vi "SPI peripheral1.vi"() -> ()   [LabVIEW 2014]
uses:
  <vilib>/Platform/TimedLoop/XDataNode/timing_clust.ctl
  <vilib>/Platform/TimedLoop/XDataNode/nitl_modes.ctl
  <vilib>/Platform/TimedLoop/XDataNode/wakeup.ctl
  <userlib>/_NI SPI IP/FPGA/Controllers/Public/Transfer Settings.ctl
  <vilib>/rvi/Emulation/niFpgaGetClockAttributes.vi
  <vilib>/rvi/Emulation/niFpgaSctlEmulationGetInTimedLoop.vi
  <vilib>/rvi/Emulation/niFpgaEmulationReportErrorSimple.vi
  <vilib>/rvi/Emulation/niFpgaCriticalErrorInLSC.vi
  <vilib>/rvi/interface/RandomDataEmulation/niFpgaRandomDataHandleErrors.vi
  <vilib>/rvi/eio/common/nirviEmuTemplateMethod_errors.vi
  <vilib>/Platform/TimedLoop/XDataNode/XDataNode.xnode
  <vilib>/rvi/DataTransferAndStorage/Container/XNode/niFpgaContainer.xnode
  <vilib>/rvi/interface/RandomDataEmulation/nirviRandomDataFpgaReadWriteTemplate.vi
  <vilib>/eio/EIONode/EIONode.xnode
  <vilib>/Platform/TimedLoop/XDataNode/XDNodeRunTimeDep.lvlib
  <userlib>/_NI SPI IP/FPGA/Controllers/NI SPI IP FPGA.lvlib
panel:
  out "Element":u32
  in  "Start/Reset":bool
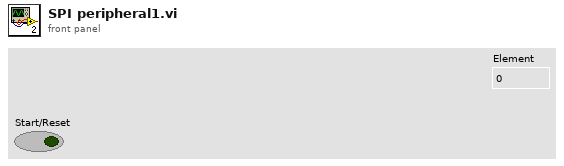
[diagram p1: front panel]
types:
  T1 = typedef "NI SPI IP FPGA.lvlib/Transfer Settings.ctl" = cluster{"Divide Value":u8, "Transfer Length (bits)":u8, "CS Asserted Polarity":bool, "Clock Polarity (CPOL)":bool, "Clock Phase (CPHA)":bool, "Lengthen MISO Setup":bool, "Direction Change Bit":u8, "MOSI Starts as Output":bool, "Tristatable MOSI":bool}
  T2 = typedef "XDNodeRunTimeDep.lvlib/timing_clust.ctl" = cluster{"Expected End [f-1]":u64, "Actual End [f-1]":u64, "Finished Late? [f-1]":bool, "Expected End [i-1]":u64, "Actual End [i-1]":u64, "Finished Late? [i-1]":bool, "Expected Start [i]":u64, "Actual Start [i]":u64, "Expected Start [f]":u64, "Actual Start [f]":u64, "Source Name":string, "Structure Name":string, "Period":i64, "Deadline":i64, "Offset":i64, "Start":i64, "Priority":i32, "Timeout":i32, "Mode":T3, "Wakeup Reason":T4, "Error":errorcluster, "Source Type":string, "Secondary Source Type":string, "Global End Time":u64, "Global Start Time":u64, "Frame Duration":u64, "Iteration Duration":u64, "Assigned CPU":i32, "I/O Scan Engine Mode":u32}
  T3 = typedef "XDNodeRunTimeDep.lvlib/nitl_modes.ctl" = enum32{"No Change", "Process missed periods, maintain original phase", "Discard missed periods, maintain original phase", "Process missed periods, ignore original phase", "Discard missed periods, ignore original phase"}
  T4 = typedef "XDNodeRunTimeDep.lvlib/wakeup.ctl" = enum32{"Normal", "Aborted", "Asynchronous wakeup", "Timing source error", "Timed loop error", "Timeout"}
  T5 = typedef "NI SPI IP FPGA.lvlib/Spi Master Outputs.ctl" = cluster{"Chip Select":bool, "Clock":bool, "MOSI":bool, "MOSI OE":bool}
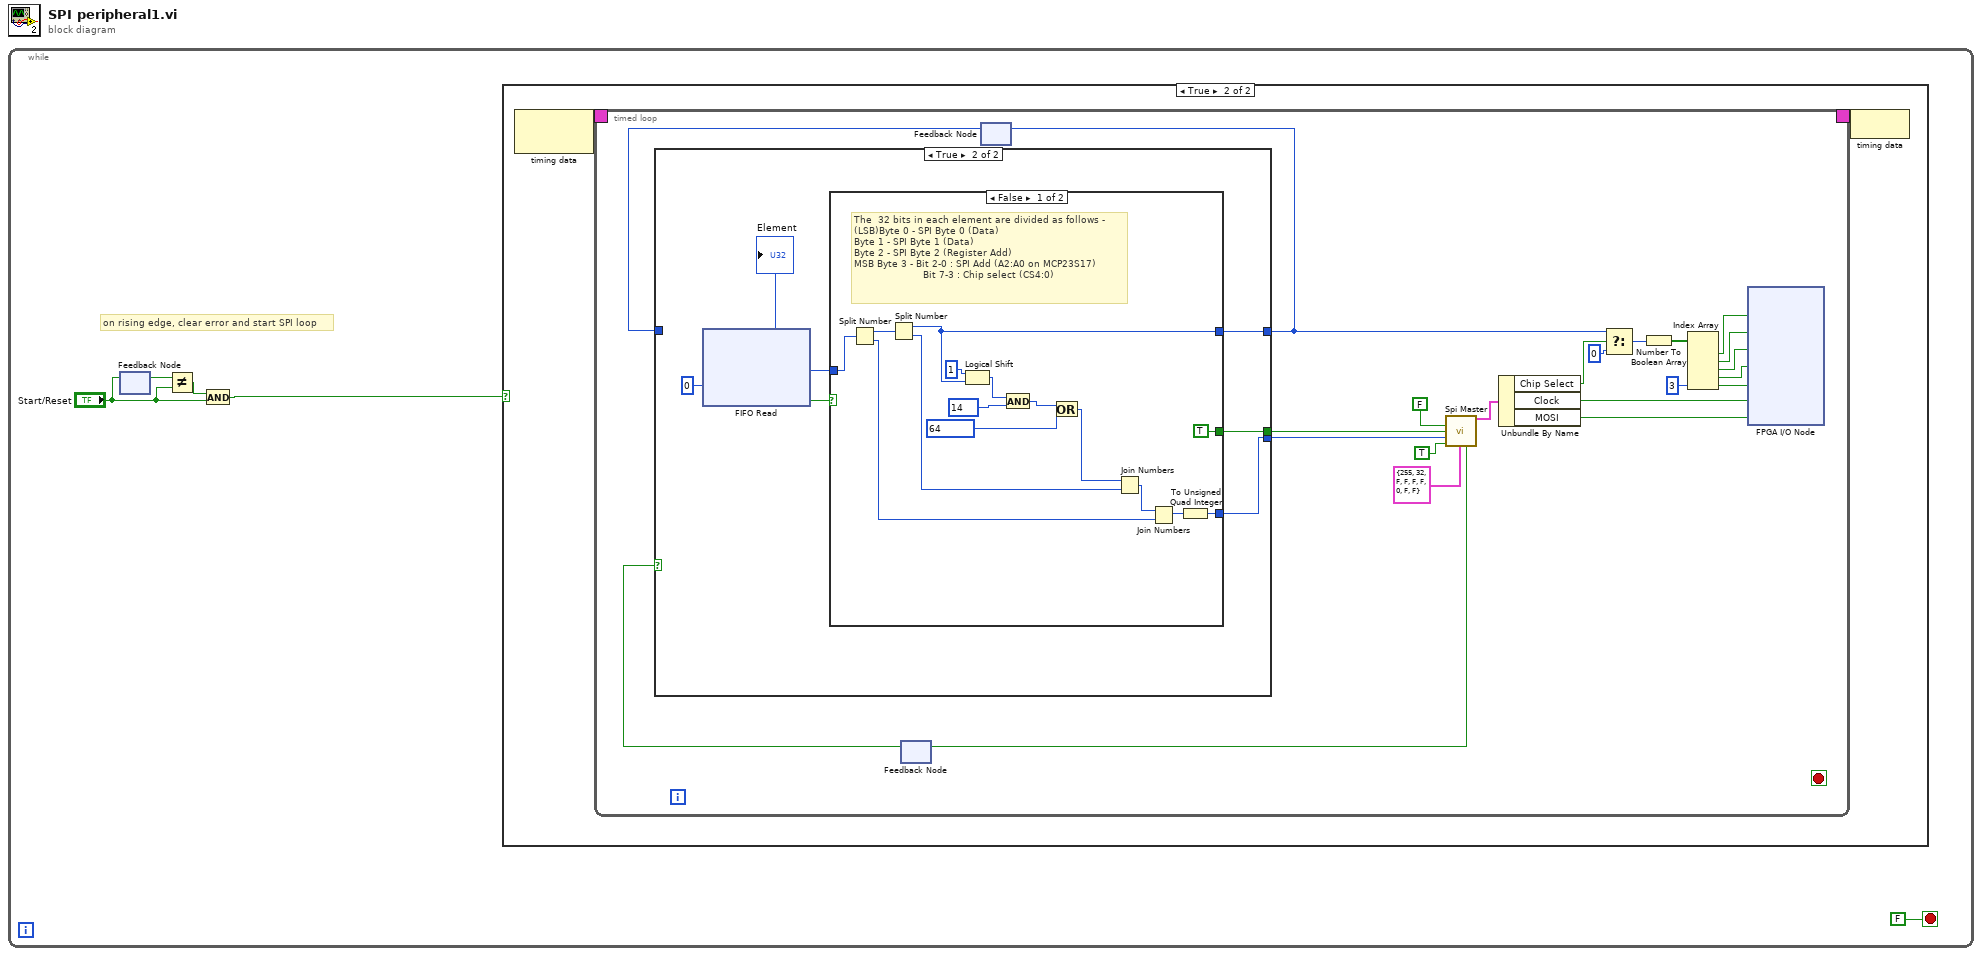
[diagram p0: block diagram]
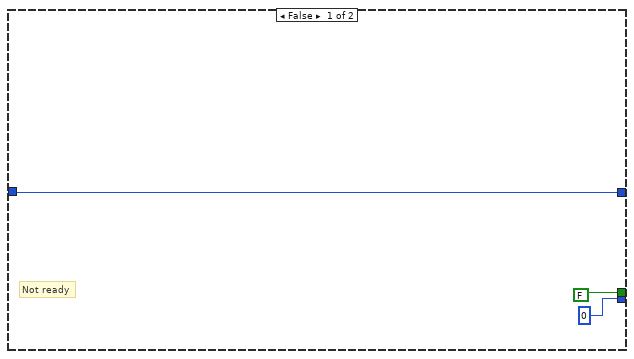
[diagram p3: hidden frame]
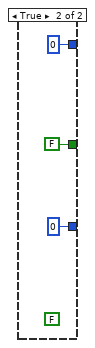
[diagram p4: hidden frame]
diagram:
  n1 = while {
    stop <- FALSE stop-if-true
    # "on rising edge, clear error and start SPI loop"
    n2 = feedback #1() -> (w4:bool)  [unwired: 1 in]
    n3 = feedback-in #1("Start/Reset") -> ()
    n4 = Not Equal?(x=w4, y="Start/Reset") -> (x != y?=w2:bool)
    n5 = And(x=w2, y="Start/Reset") -> (x .and. y?=w1:bool)
    n6 = case shown="True" w1 {
      frame False {
      }
      frame True {
        n7 = node-c288() -> (w7:T2)  [unwired: 1 in]
        n8 = timed-loop {
          timing: w7 -> [_]
          timing-out: [_] -> w6
          stop <- _ stop-if-true
          n9 = feedback #2() -> (w13:bool)  [unwired: 1 in]
          n10 = feedback #3() -> (w10:u8)  [unwired: 1 in]
          n11 = case shown="True" w13 {
            tunnel: [w30 w38] -> w11
            tunnel: [u64 0 w37] -> w9
            tunnel: [FALSE ("start strobe") w36] -> w12
            tunnel: w10 -> [w30 _]
            frame False {
              # "Not ready"
            }
            frame True {
              n12 = xnode ("FIFO Read")("Timeout"=0) -> ("Element"=w34:u32, "Timed Out?"=w33:bool)  [unwired: 1 in, 1 out]
              "Element" <- w34
              n13 = case shown="False" w33 {
                tunnel: w34 -> [w53 _]
                tunnel: [w42 u8 0] -> w38
                tunnel: [w40 u64 0] -> w37
                tunnel: [TRUE ("manual assert chip select") FALSE ("manual assert chip select")] -> w36
                frame False {
                  # "The  32 bits in each element are divided as follows -\n(LSB)Byte 0 - SPI Byte 0 (Data)\nByte 1 - SPI Byte 1 (Data)\nByte 2 - SPI Byte 2 (Register Add)\nMSB Byte 3 - Bit 2-0 : SPI Add (A2:A0 on MCP23S17)\n                       Bit 7-3 : Chip select (CS4:0)"
                  n14 = Split Number(x=w53) -> (hi(x)=w52:u16, lo(x)=w46:u16)
                  n15 = Split Number(x=w52) -> (hi(x)=w42:u8, lo(x)=w48:u8)
                  n16 = Logical Shift(y=i16 1, x=w42) -> (x << y=w50:u8)
                  n17 = And(x=w50, y=u8 14) -> (x .and. y?=w45:u8)
                  n18 = Or(x=w45, y=u8 64) -> (x .or. y?=w43:u8)
                  n19 = Join Numbers(hi=w43, lo=w48) -> ((hi.lo)=w47:u16)
                  n20 = Join Numbers(hi=w47, lo=w46) -> ((hi.lo)=w41:u32)
                  n21 = To Unsigned Quad Integer(1:w41) -> (0:w40:u64)
                }
                frame True {
                  (unwired) FALSE
                }
              }
            }
          }
          n22 = feedback-in #3(w11) -> ()
          n23 = call <userlib>:"Spi Master.vi"("manual assert chip select"=FALSE, "start strobe"=w12, "data to write"=w9, "MOSI output enable done"=TRUE, "spi transfer settings"=T1 {"Divide Value"=255, "Transfer Length (bits)"=32, "CS Asserted Polarity"=FALSE, "Clock Polarity (CPOL)"=FALSE, "Clock Phase (CPHA)"=FALSE, "Lengthen MISO Setup"=FALSE, "Direction Change Bit"=0, "MOSI Starts as Output"=FALSE, "Tristatable MOSI"=FALSE}) -> ("spi output"=w25:T5, "ready for input"=w14:bool)  [unwired: 7 in, 2 out]
          n24 = feedback-in #2(w14) -> ()
          n25 = Unbundle By Name(w25) -> ("Chip Select"=w24:bool, "Clock"=w17:bool, "MOSI"=w16:bool)
          n26 = Select(t=w11, s=w24, f=u8 0) -> (s? t:f=w15:u8)
          n27 = Number To Boolean Array(number=w15) -> (Boolean array=w29:bool[])
          n28 = Index Array(array=w29, index #5=3 ("index")) -> (element #1=w28:bool, element #2=w21:bool, element #3=w20:bool, element #4=w19:bool, element #5=w18:bool)  [unwired: 4 in]
          n29 = xnode "FPGA I/O Node"("CS4"=w28, "CS3"=w21, "CS2"=w20, "CS1"=w19, "CS0"=w18, "SCLK"=w17, "MOSI"=w16) -> ()  [unwired: 7 in, 7 out]
        }
        n30 = node-c288(w6) -> ()
      }
    }
  }
